vi "Buttons.vi"() -> ()   [LabVIEW 2010]
panel:
  in  "System Save Button":bool
  in  "System Refresh Button":bool
  in  "System Print Button":bool
  in  "System Pause Button":bool
  in  "System Open Button":bool
  in  "System OK Button":bool
  in  "System Load Button":bool
  in  "System Info Button":bool
  in  "System Cancel Button":bool
  in  "System Email Button":bool
  in  "System Next Button":bool
  in  "System Back Button":bool
  # "Buttons"
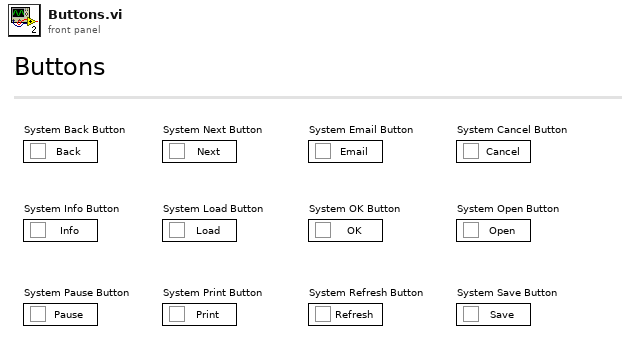
[diagram p1: front panel]
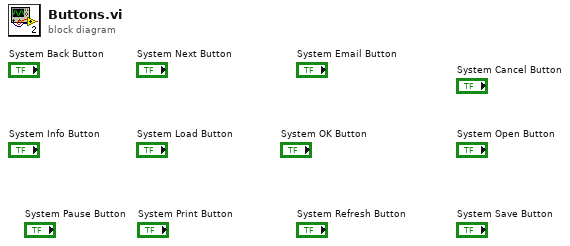
[diagram p0: block diagram]
diagram:
